vi "SetPID_ESP.vi"(0 "VISA resource name":refnum<visa-resource-name>, 2 "Axis":u16=2) -> (5 "VISA resource name out":refnum<visa-resource-name>)   [LabVIEW 2022 SP3]
uses:
  <instrlib>/Newport ESP301/Newport ESP301.lvlib
panel:
  in  "Max Accel":dbl=400.0
  in  "Max Vel":dbl=40.0
  out "error out":errorcluster
  in  "error in (no error)":errorcluster
  in  "Following Error (FE)":i32=30000
  in  "Derivative (KD)":i32=530
  in  "Integral (KI)":i32=150
  in  "Gain (KP)":i32=240
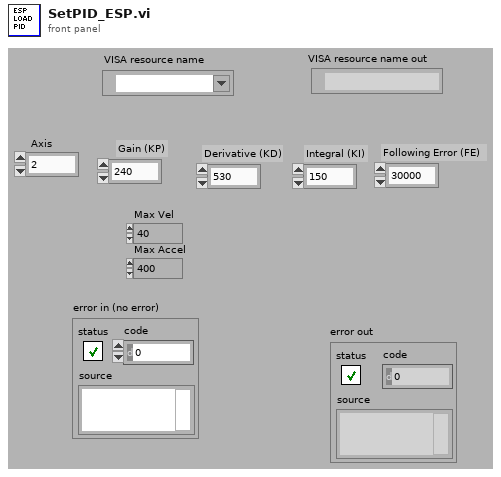
[diagram p1: front panel]
types:
  T1 = enum16{"Encoder Count", "Motor Step", "millimeter", "micrometer", "inch", "milli-inch", "micro-inch", "degree", "gradian", "radian", "milliradian", "microradian"}
  T2 = cluster{"enable Hardware limit error checking":bool, "disable motor on Hardware limit error event":bool, "abort motion on Hardware limit error event":bool, "reserved":bool, "reserved":bool, "hardware limit input (F:active low, T:active high)":bool, "reserved  ":bool, "reserved":bool, "reserved  ":bool, bool, "reserved":bool, "reserved":bool, "reserved ":bool, "reserved ":bool, "reserved":bool, "reserved ":bool, "reserved":bool, "reserved ":bool, "reserved ":bool, "reserved ":bool, "reserved ":bool, "reserved ":bool, "reserved ":bool, "reserved ":bool, "reserved ":bool, "reserved ":bool, "reserved ":bool, "reserved ":bool, "reserved ":bool, "reserved ":bool, "reserved ":bool, "reserved":bool}
  T3 = cluster{"enable motor following error checking":bool, "disable motor power on following error event":bool, "abort motion on following error event":bool, "reserved":bool, "reserved":bool, "reserved  ":bool, "reserved  ":bool, "reserved  ":bool, "reserved  ":bool, bool, "reserved":bool, "reserved":bool, "reserved ":bool, "reserved ":bool, "reserved":bool, "reserved ":bool, "reserved":bool, "reserved ":bool, "reserved ":bool, "reserved ":bool, "reserved ":bool, "reserved ":bool, "reserved ":bool, "reserved ":bool, "reserved ":bool, "reserved ":bool, "reserved ":bool, "reserved ":bool, "reserved ":bool, "reserved ":bool, "reserved ":bool, "reserved":bool}
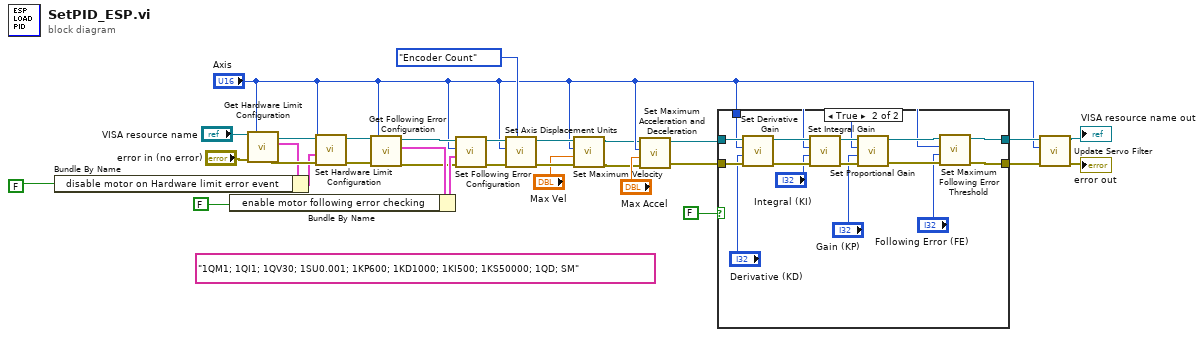
[diagram p0: block diagram]
diagram:
  (unwired) "1QM1; 1QI1; 1QV30; 1SU0.001; 1KP600; 1KD1000; 1KI500; 1KS50000; 1QD; SM"
  n1 = call <instrlib>:"Get Hardware Limit Configuration.vi"("error in (no error)"="error in (no error)", "Axis (1)"="Axis", "VISA resource name"="VISA resource name") -> ("error out"=w12:errorcluster, "Harware limit Configuration"=w11:T2, "VISA resource name out"=w13:refnum<visa-resource-name>)  [unwired: 2 in]
  n2 = Bundle By Name(cluster=w11, "disable motor on Hardware limit error event"=FALSE) -> (w9:T2)
  n3 = call <instrlib>:"Set Hardware Limit Configuration.vi"("error in (no error)"=w12, "Harware limit Configuration"=w9, "Axis (1)"="Axis", "VISA resource name"=w13) -> ("error out"=w15:errorcluster, "VISA resource name out"=w14:refnum<visa-resource-name>)  [unwired: 2 in]
  n4 = call <instrlib>:"Get Following Error Configuration.vi"("error in (no error)"=w15, "Axis (1)"="Axis", "VISA resource name"=w14) -> ("error out"=w18:errorcluster, "Following Error Configuration"=w20:T3, "VISA resource name out"=w19:refnum<visa-resource-name>)  [unwired: 2 in]
  n5 = Bundle By Name(cluster=w20, "enable motor following error checking"=FALSE) -> (w22:T3)
  n6 = call <instrlib>:"Set Following Error Configuration.vi"("error in (no error)"=w18, "Following Error Configuration"=w22, "Axis (1)"="Axis", "VISA resource name"=w19) -> ("error out"=w16:errorcluster, "VISA resource name out"=w17:refnum<visa-resource-name>)  [unwired: 2 in]
  n7 = call <instrlib>:"Set Axis Displacement Units.vi"("Units (Encoder Count)"=T1."Encoder Count", "error in (no error)"=w16, "Axis (1)"="Axis", "VISA resource name"=w17) -> ("error out"=w25:errorcluster, "VISA resource name out"=w26:refnum<visa-resource-name>)  [unwired: 3 in]
  n8 = call <instrlib>:"Set Maximum Velocity.vi"("error in (no error)"=w25, "Maximum Velocity (0 units/s)"="Max Vel", "Axis (1)"="Axis", "VISA resource name"=w26) -> ("error out"=w3:errorcluster, "VISA resource name out"=w4:refnum<visa-resource-name>)  [unwired: 2 in]
  n9 = call <instrlib>:"Set Maximum Acceleration and Deceleration.vi"("error in (no error)"=w3, "Acceleration (0 units/s²)"="Max Accel", "Axis (1)"="Axis", "VISA resource name"=w4) -> ("error out"=w1:errorcluster, "VISA resource name out"=w2:refnum<visa-resource-name>)  [unwired: 2 in]
  n10 = case shown="True" FALSE {
    tunnel: w2 -> [w33 w48]
    tunnel: w1 -> [w32 w45]
    tunnel: [w33 w36] -> w24
    tunnel: [w32 w35] -> w23
    tunnel: "Axis" -> [_ w34]
    frame False {
    }
    frame True {
      n11 = call <instrlib>:"Set Derivative Gain.vi"("error in (no error)"=w45, "Kd (0)"="Derivative (KD)", "Axis (1)"=w34, "VISA resource name"=w48) -> ("error out"=w44:errorcluster, "VISA resource name out"=w47:refnum<visa-resource-name>)  [unwired: 2 in]
      n12 = call <instrlib>:"Set Integral Gain.vi"("error in (no error)"=w44, "Ki (0)"="Integral (KI)", "Axis (1)"=w34, "VISA resource name"=w47) -> ("error out"=w43:errorcluster, "VISA resource name out"=w46:refnum<visa-resource-name>)  [unwired: 2 in]
      n13 = call <instrlib>:"Set Proportional Gain.vi"("error in (no error)"=w43, "Kp (0)"="Gain (KP)", "Axis (1)"=w34, "VISA resource name"=w46) -> ("error out"=w38:errorcluster, "VISA resource name out"=w39:refnum<visa-resource-name>)  [unwired: 2 in]
      n14 = call <instrlib>:"Set Maximum Following Error Threshold.vi"("error in (no error)"=w38, "Maximum error allowed (0 units)"="Following Error (FE)", "Axis (1)"=w34, "VISA resource name"=w39) -> ("error out"=w35:errorcluster, "VISA resource name out"=w36:refnum<visa-resource-name>)  [unwired: 2 in]
    }
  }
  n15 = call <instrlib>:"Update Servo Filter.vi"("error in (no error)"=w23, "Axis (0)"="Axis", "VISA resource name"=w24) -> ("error out"=→"error out":errorcluster, "VISA resource name out"=→"VISA resource name out":refnum<visa-resource-name>)  [unwired: 3 in]
